vi "Inst.KH7008.getChassis.vi"(8 "error in (no error)":errorcluster, 11 "Inst.Krohn-Hite-7008 in":refnum<class "Inst.Krohn-Hite-7008.lvclass">) -> (0 "error out":errorcluster, 2 "Number of Chassis":i32, 3 "Inst.Krohn-Hite-7008 out":refnum<class "Inst.Krohn-Hite-7008.lvclass">)   [LabVIEW 2019, in "Inst.KH7008.lvlib" / "Inst.Krohn-Hite-7008.lvclass"]
doc: "Returns the installed shunt resistor set"
uses:
  Inst.Krohn-Hite-7008.lvclass
  1fdc1f3d-332e-4594-8a59-3c61ed5849a6.vi
  Typedefs/Inst.KH7008.Commands--Enum.ctl
  Typedefs/getChassisResponse--Cluster.ctl
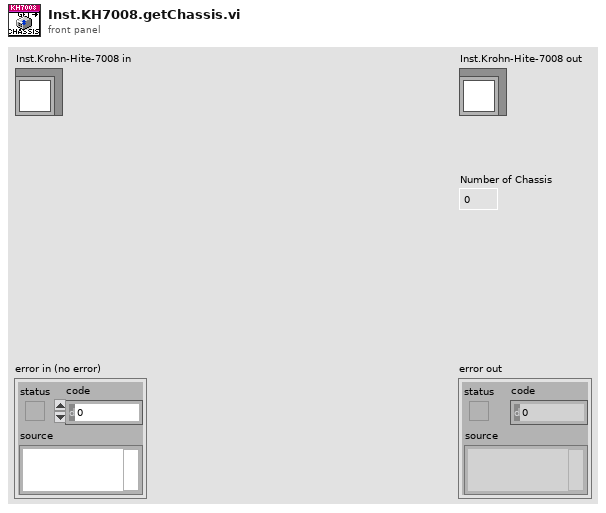
[diagram p1: front panel]
types:
  T1 = typedef "Inst.KH7008.lvlib/Inst.Krohn-Hite-7008.lvclass/getChassisResponse--Cluster.ctl" = cluster{"Chassis":i32}
  T2 = typedef "Inst.KH7008.lvlib/Inst.Krohn-Hite-7008.lvclass/Inst.KH7008.Commands--Enum.ctl" = enum16{"getChannel", "getAllChannels", "setChannel", "setAllChannels", "getShuntResistor", "getChassis"}
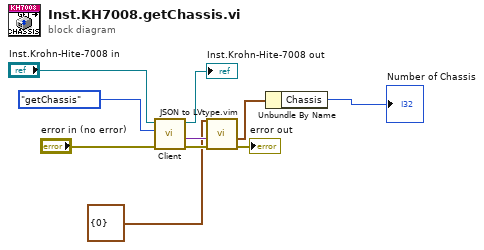
[diagram p0: block diagram]
diagram:
  n1 = call-dynamic "Client.vi"("error in (no error)"="error in (no error)", "Command in"=Inst.KH7008.Commands--Enum."getChassis" ("publicCommands"), "Instrument in"="Inst.Krohn-Hite-7008 in") -> ("error out"=w5:errorcluster, "Data out"=w6:variant, "Instrument out"=→"Inst.Krohn-Hite-7008 out":refnum<class "Inst.Krohn-Hite-7008.lvclass">)  [unwired: 5 in, 1 out]
  n2 = call "JSON to LVtype.vim"("type"=T1 {"Chassis"=0} ("getChassis"), "error in (no error)"=w5, "JSON Data in"=w6) -> ("error out"=→"error out":errorcluster, "Data out"=w3:T1)  [unwired: 7 in]
  n3 = Unbundle By Name(w3) -> ("Chassis"=→"Number of Chassis":i32)
